vi "create queues External.vi"(8 "error in (no error)":errorcluster) -> (0 "error out":errorcluster)   [LabVIEW 2026]
uses:
  image.ctl
  Automotive Vision.lvclass
panel:
  in  "stop":bool
  out "element":T1
  out "# elements in queue":i32
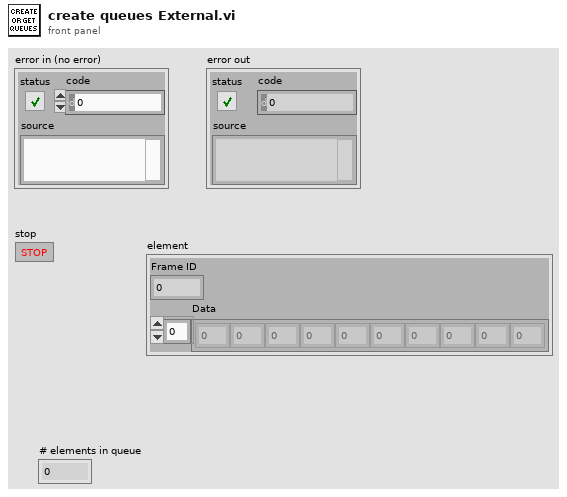
[diagram p1: front panel]
types:
  T1 = typedef "Automotive Vision.lvclass/image.ctl" = cluster{"Frame ID":u32, "Data":u8[]}
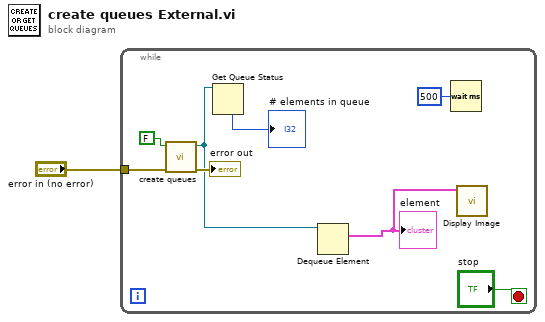
[diagram p0: block diagram]
diagram:
  n1 = while {
    tunnel: "error in (no error)" -> [w8]
    stop <- "stop" stop-if-true
    n2 = call "create queues.vi"("error in (no error)"=w8, "create if not found? (T)"=FALSE) -> ("error out"=→"error out":errorcluster, "image queue out"=w5:refnum<queue>)  [unwired: 5 in, 3 out]
    n3 = Get Queue Status(queue=w5) -> (# elements in queue=→"# elements in queue":i32)  [unwired: 2 in, 7 out]
    n4 = Dequeue Element(queue=w5) -> (element=w2:T1)  [unwired: 2 in, 3 out]
    "element" <- w2
    n5 = Wait (ms)(milliseconds to wait=u32 500) -> ()  [unwired: 1 out]
    n6 = call "Display Image.vi"("Data"=w2) -> ()  [unwired: 11 in]
  }
